vi "Teleop.vi"(10 "Match Info":T1={"Autonomous Elapsed Seconds"=0.0, "TeleOp Elapsed Seconds"=0.0, "Disabled Elapsed Seconds"=0.0, "Visited Autonomous"=FALSE, "Visited TeleOp"=FALSE, "Visited Disabled"=FALSE, "Autonomous Settings"={"Autonomous Style"=enum."Independent", "VI Refnum"=refnum}}, 11 "Call Context":T2) -> ()   [LabVIEW 2015]
doc: "This VI is called for each enabled TeleOp packet received from the DS. It is typically used to read from joysticks and other inputs and update I/O or setpoints for timed control loops. It should complete and return within 20 milliseconds or risk missing DS packets."
uses:
  <vilib>/Rock Robotics/WPI/DriverStation/WPI_DriverStationDerivedRobotMode.ctl
  <vilib>/Rock Robotics/WPI/DriverStation/WPI_DriverStationMatch Info.ctl
  <vilib>/Rock Robotics/WPI/Utilities/WPI_GetSetVariantRefNum.vi
  <vilib>/Rock Robotics/Network Tables/NT Write Boolean Array.vi
  <vilib>/Rock Robotics/Network Tables/NT Write Numeric Array.vi
  Framework/Robot Global Data.vi
  <vilib>/Rock Robotics/Network Tables/NT Write Number.vi
  <vilib>/Rock Robotics/Network Tables/NT Write Boolean.vi
panel:
  in  "Setpoint":dbl
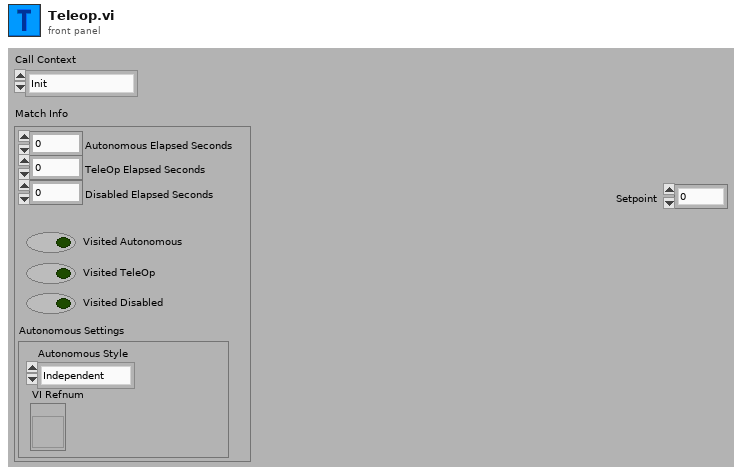
[diagram p1: front panel]
types:
  T1 = typedef "WPI_DriverStationMatch Info.ctl" = cluster{"Autonomous Elapsed Seconds":dbl, "TeleOp Elapsed Seconds":dbl, "Disabled Elapsed Seconds":dbl, "Visited Autonomous":bool, "Visited TeleOp":bool, "Visited Disabled":bool, "Autonomous Settings":cluster{"Autonomous Style":enum16{"Iterative", "Independent"}, "VI Refnum":refnum<vi>}}
  T2 = typedef "WPI_DriverStationDerivedRobotMode.ctl" = enum16{"Init", "Execute", "Stop"}
  T3 = typedef "WPI_MotorControlDeviceRef.ctl" = cluster{"DeviceStatus":errorcluster, "Type":T4, "PWM":cluster{"PWM Channel":T5, "DeadBand":T6}, "CAN":cluster{"Device Number":u8, "Control Mode":T7, "Semaphore":T8, "Max Vout":dbl, "TalonSRX Control Mode":T9}, "Invert":bool}
  T4 = typedef "WPI_MotorControlType.ctl" = enum16{"PWM", "CAN", "CANTalonSRX"}
  T5 = typedef "FPGA_DIOPWMChannel.ctl" = enum8{"PWM 0", "PWM 1", "PWM 2", "PWM 3", "PWM 4", "PWM 5", "PWM 6", "PWM 7", "PWM 8", "PWM 9", "PWM MXP 0", "PWM MXP 1", "PWM MXP 2", "PWM MXP 3", "PWM MXP 4", "PWM MXP 5", "PWM MXP 6", "PWM MXP 7", "PWM MXP 8", "PWM MXP 9", "Invalid"}
  T6 = typedef "WPI_PWMDeadband.ctl" = cluster{"Name":string, "maxPositivePwm":i32, "minPositivePwm":i32, "centerPwm":i32, "maxNegativePwm":i32, "minNegativePwm":i32, "angularRange":u16}
  T7 = typedef "WPI_CANJaguar_ControlMode.ctl" = enum8{"Percent VBus", "Current", "Speed", "Position", "Voltage"}
  T8 = typedef "Semaphore RefNum" = refnum<k1>
  T9 = typedef "WPI_CANTalonSRX_APIControlMode.ctl" = enum8{"Percent VBus", "Speed", "Position", "Slave", "Unchanged / Invalid", "Voltage Compensation", "Current", "Motion Profile"}
  T10 = typedef "WPI_CANTalonSRX_GlobalStatus.ctl" = cluster{"Applied Throttle":dbl, "Module Enabled":bool, "CAN Error":errorcluster, "Closed Loop Error":dbl, "Forward Limit Switch Closed":bool, "Reverse Limit Switch Closed":bool, "Sensor Position":dbl, "Sensor Velocity":dbl, "Current":dbl, "Sticky Fault - Over Temp":bool, "Sticky Fault - Under Voltage":bool, "Sticky Fault - Forward Limit":bool, "Sticky Fault - Reverse Limit":bool, "Sticky Fault - Forward Soft Limit":bool, "Sticky Fault - Reverse Soft Limit":bool, "Brake is Enabled":bool, "Encoder Position":dbl, "Encoder Velocity":dbl, "Encoder Index Count":dbl, "Encoder A Pin State":bool, "Encoder B Pin State":bool, "Encoder Index Pin State":bool, "Analog In":dbl, "Analog In Velocity":dbl, "Temperature (C)":dbl, "Battery Voltage":dbl, "Control 5 Is Supported":bool, "Current Profile Slot Select":dbl, "Pos Div 8":bool, "Vel Div 4":bool, "Pulse Width Position":i32, "Pulse Width Velocity":i32, "Pulse Width Rise To Rise (us)":i32, "Pulse Width Rise To Fall (us)":i32, "Mot Prof Active Is Under Run":bool, "Mot Prof Active Has Under Run":bool, "Mot Prof Active Is Last":bool, "Mot Prof Active Velocity Only":bool, "Mot Prof Active Is Valid":bool, "Mot Prof Buffer Is Full":bool, "Mot Prof Active Profile Slot Select":i32, "Mot Prof NextID":i32, "Mot Prof Count":i32, "Mot Prof Active Velocity":dbl, "Mot Prof Active Position":dbl, "Mot Prof Output Enable":i32}
  T11 = typedef "WPI_JoystickDevRef.ctl" = cluster{"Device":T12}
  T12 = typedef "WPI_JoystickDeviceEnum.ctl" = enum16{"USB 0", "USB 1", "USB 2", "USB 3", "USB 4", "USB 5"}
  T13 = typedef "WPI_AnalogChannelDevRef.ctl" = cluster{"DevStatus":errorcluster, "Analog Channel":T14}
  T14 = typedef "FPGA_AIChannel.ctl" = enum8{"AI 0", "AI 1", "AI 2", "AI 3", "AI MXP 0", "AI MXP 1", "AI MXP 2", "AI MXP 3", "Invalid"}
  T15 = typedef "WPI_CompressorDevRef.ctl" = cluster{"DevStatus":errorcluster, "Pneumatics Control Module":u8}
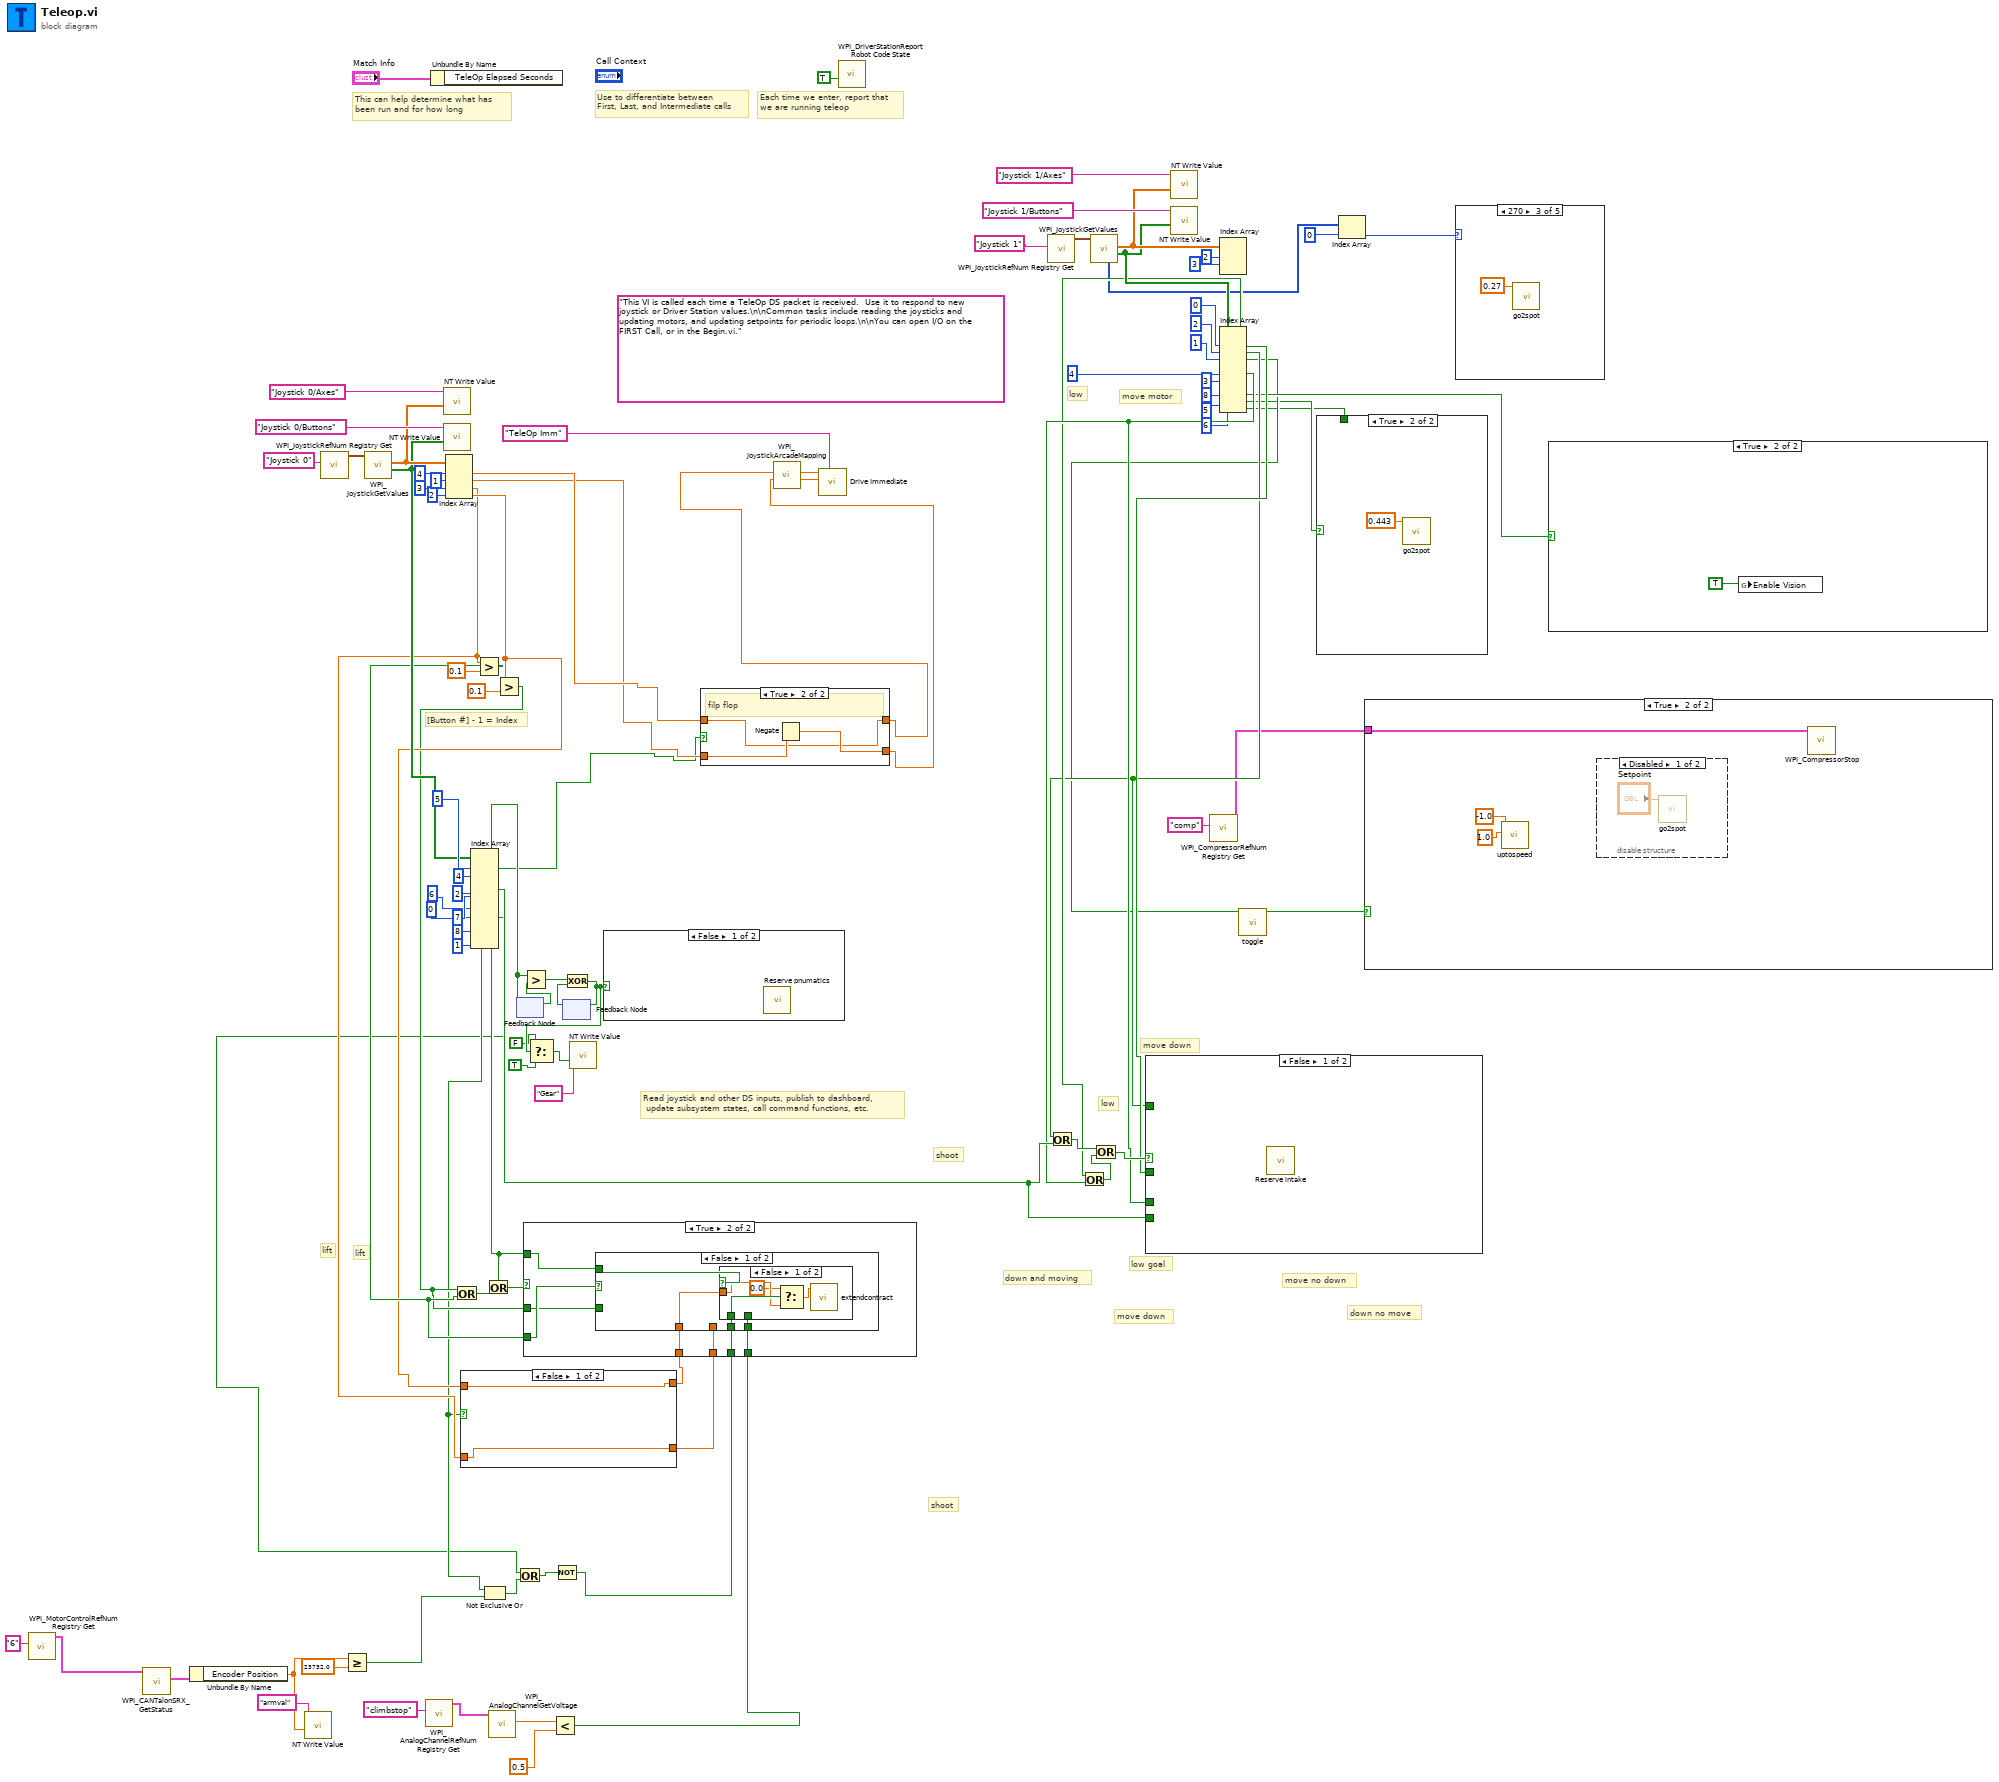
[diagram p0: block diagram]
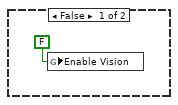
[diagram p2: hidden frame]
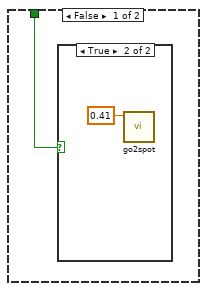
[diagram p3: hidden frame]
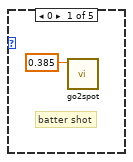
[diagram p5: hidden frame]
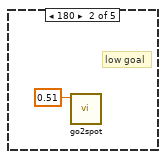
[diagram p6: hidden frame]
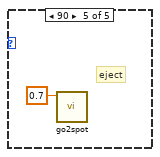
[diagram p8: hidden frame]
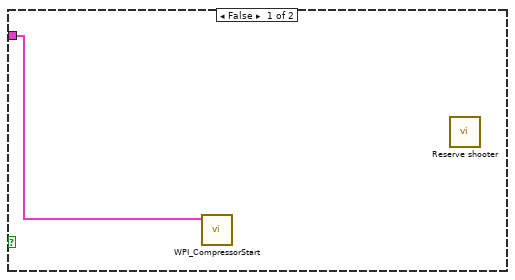
[diagram p9: hidden frame]
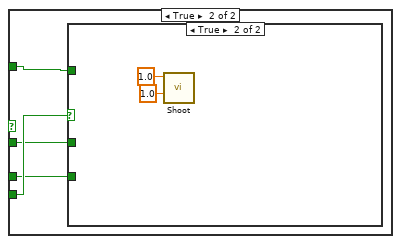
[diagram p12: hidden frame]
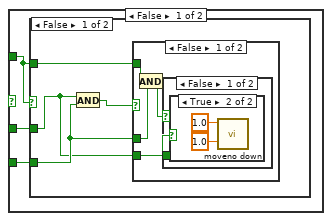
[diagram p13: hidden frame]
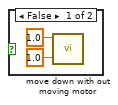
[diagram p14: hidden frame]
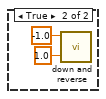
[diagram p15: hidden frame]
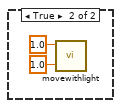
[diagram p16: hidden frame]
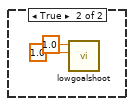
[diagram p17: hidden frame]
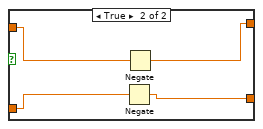
[diagram p18: hidden frame]
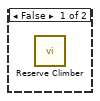
[diagram p19: hidden frame]
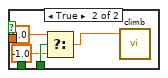
[diagram p20: hidden frame]
diagram:
  (unwired) "This VI is called each time a TeleOp DS packet is received.  Use it to respond to new joystick or Driver Station values.\n\nCommon tasks include reading the joysticks and updating motors, and updating setpoints for periodic loops.\n\nYou can open I/O on the FIRST Call, or in the Begin.vi."
  # "move down"
  # "low"
  # "down no move"
  # "move no down"
  # "shoot"
  # "low goal"
  # "down and moving"
  # "move down"
  # "shoot"
  # "move motor"
  # "low"
  # "lift"
  # "lift"
  # "[Button #] - 1 = Index"
  # "Read joystick and other DS inputs, publish to dashboard,\n update subsystem states, call command functions, etc."
  # "Each time we enter, report that\nwe are running teleop"
  # "Use to differentiate between\nFirst, Last, and Intermediate calls"
  # "This can help determine what has\nbeen run and for how long"
  n1 = call <vilib>:"WPI_MotorControlRefNum Registry Get.vi"("refnum name"="6") -> ("MotorControlDevRef"=w17:T3)  [unwired: 9 in, 1 out]
  n2 = call <vilib>:"WPI_CANTalonSRX_GetStatus.vi"("CAN Talon SRX Ref"=w17) -> ("Talon SRX Status"=w16:T10)  [unwired: 8 in, 2 out]
  n3 = Unbundle By Name(w16) -> ("Encoder Position"=w2:dbl)
  n4 = call-poly <vilib>:"NT Write Value.vi"("Numeric"=w2, "Name"="armval") -> ()  [unwired: 9 in, 1 out]
  n5 = call <vilib>:"WPI_JoystickRefNum Registry Get.vi"("refnum name"="Joystick 0") -> ("JoystickDevRef"=w95:T11)  [unwired: 1 in, 9 out]
  n6 = Greater Or Equal?(x=w2, y=23732.0) -> (x >= y?=w11:bool)
  n7 = call <vilib>:"WPI_JoystickGetValues.vi"("JoystickDevRef"=w95) -> ("Buttons"=w71:bool[], "Axes"=w92:dbl[])  [unwired: 6 in, 3 out]
  n8 = call <vilib>:"WPI_AnalogChannelRefNum Registry Get.vi"("refnum name"="climbstop") -> ("AIDeviceRef"=w4:T13)  [unwired: 9 in, 1 out]
  n9 = Unbundle By Name("Match Info") -> ()  [unwired: 1 out]
  n10 = call-poly <vilib>:"NT Write Value.vi"("Numeric Array"=w92, "Name"="Joystick 0/Axes") -> ()  [unwired: 9 in, 1 out]
  n11 = call-poly <vilib>:"NT Write Value.vi"("Boolean Array"=w71, "Name"="Joystick 0/Buttons") -> ()  [unwired: 9 in, 1 out]
  n12 = Index Array(array=w92, index #1=4 ("index"), index #2=1 ("index"), index #3=3 ("index"), index #4=2 ("index")) -> (element #1=w40:dbl, element #2=w39:dbl, element #3=w57:dbl, element #4=w58:dbl)
  n13 = Index Array(array=w71, index #1=5 ("index"), index #2=4 ("index"), index #4=2 ("index"), index #5=0 ("index"), index #6=6 ("index"), index #8=7 ("index"), index #10=8 ("index"), index #12=1 ("index")) -> (element #1=w38:bool, element #2=w75:bool, element #4=w49:bool, element #5=w60:bool, element #6=w10:bool, element #8=w8:bool)  [unwired: 4 in, 6 out]
  n14 = case shown="False" w10 {
    tunnel: [w100 w101] -> w56
    tunnel: w58 -> [w100 w104]
    tunnel: w57 -> [w99 w103]
    tunnel: [w99 w102] -> w3
    frame False {
    }
    frame True {
      n15 = Negate(x=w103) -> (-x=w102:dbl)
      n16 = Negate(x=w104) -> (-x=w101:dbl)
    }
  }
  n17 = Greater?(x=w57, y=0.1) -> (0:w63:bool)
  n18 = Not Exclusive Or(1:w11, 2:w10) -> (0:w9:bool)
  n19 = call <vilib>:"WPI_AnalogChannelGetVoltage.vi"("AIDeviceRef"=w4) -> ("Voltage"=w15:dbl)  [unwired: 8 in, 2 out]
  n20 = Greater?(x=w58, y=0.1) -> (0:w19:bool)
  n21 = Or(x=w19, y=w63) -> (x .or. y?=w61:bool)
  n22 = Or(x=w60, y=w61) -> (x .or. y?=w59:bool)
  n23 = feedback-in #1(w75) -> ()
  n24 = feedback #1() -> (w88:bool)  [unwired: 1 in]
  n25 = Or(x=w8, y=w9) -> (x .or. y?=w7:bool)
  n26 = Greater?(x=w75, y=w88) -> (0:w87:bool)
  n27 = Less?(x=w15, y=0.5 ("x")) -> (x < y?=w13:bool)
  n28 = Not(x=w7) -> (.not. x?=w6:bool)
  n29 = case shown="True" w59 {
    tunnel: w63 -> [_ w111]
    tunnel: w3 -> [_ w110]
    tunnel: w56 -> [_ w109]
    tunnel: w60 -> [_ w108]
    tunnel: w13 -> [_ w107]
    tunnel: w19 -> [_ w106]
    tunnel: w6 -> [_ w105]
    frame False {
      n30 = call "Reserve Climber.vi"() -> ()  [unwired: 11 in, 1 out]
    }
    frame True {
      n31 = case shown="False" w111 {
        tunnel: w110 -> [_ w125]
        tunnel: w109 -> [w115 w124]
        tunnel: w108 -> [w114 _]
        tunnel: w107 -> [w113 _]
        tunnel: w106 -> [_ w126]
        tunnel: w105 -> [w112 _]
        frame False {
          n32 = case shown="False" w114 {
            tunnel: w115 -> [w118 _]
            tunnel: w113 -> [_ w123]
            tunnel: w112 -> [w119 _]
            frame False {
              n33 = Select(t=0.0, s=w119, f=w118) -> (s? t:f=w116:dbl)
              n34 = call "extendcontract.vi"("Setpoint"=w116) -> ()  [unwired: 10 in, 1 out]
            }
            frame True {
              n35 = Select(t=0.0, s=w123, f=-1.0) -> (s? t:f=w120:dbl)
              n36 = call "climb.vi"("Setpoint"=w120) -> ()  [unwired: 10 in, 1 out]
            }
          }
        }
        frame True {
          n37 = case shown="True" w126 {
            tunnel: w125 -> [w127 w128]
            tunnel: w124 -> [_ w129]
            frame False {
              n38 = call "liftlower.vi"("Setpoint"=w127) -> ()  [unwired: 10 in, 1 out]
            }
            frame True {
              n39 = call "lift and contract.vi"("lift"=w128, "Setpoint"=w129) -> ()  [unwired: 9 in, 1 out]
            }
          }
        }
      }
    }
  }
  n40 = feedback #2() -> (w86:bool)  [unwired: 1 in]
  n41 = Exclusive Or(1:w86, 2:w87) -> (0:w43:bool)
  n42 = Select(t=FALSE, s=w43, f=TRUE) -> (s? t:f=w35:bool)
  n43 = feedback-in #2(w43) -> ()
  n44 = call-poly <vilib>:"NT Write Value.vi"("Boolean"=w35, "Name"="Gear") -> ()  [unwired: 9 in, 1 out]
  n45 = case shown="False" w43 {
    frame False {
      n46 = call "Reserve pnumatics.vi"() -> ()  [unwired: 11 in, 1 out]
    }
    frame True {
      n47 = call "Activate Da intake.vi"("Setpoint"=1.0) -> ()  [unwired: 10 in, 1 out]
    }
  }
  n48 = case shown="True" w38 {
    tunnel: w39 -> [w131 w135]
    tunnel: [w131 w134] -> w41
    tunnel: w40 -> [w132 w133]
    tunnel: [w132 w133] -> w42
    frame False {
    }
    frame True {
      # "filp flop"
      n49 = Negate(x=w135) -> (-x=w134:dbl)
    }
  }
  n50 = call <vilib>:"WPI_JoystickArcadeMapping.vi"("Y axis value"=w41, "X axis value"=w42) -> ("Right Motor Value"=w84:dbl, "Left Motor Value"=w85:dbl)  [unwired: 8 in]
  n51 = call "Drive Immediate.vi"("Description"="TeleOp Imm", "Right Setpoint"=w84, "Left Setpoint"=w85) -> ()  [unwired: 8 in, 1 out]
  n52 = call <vilib>:"WPI_DriverStationReport Robot Code State.vi"("TeleOp"=TRUE ("Autonomous")) -> ()  [unwired: 10 in, 1 out]
  n53 = call <vilib>:"WPI_JoystickRefNum Registry Get.vi"("refnum name"="Joystick 1") -> ("JoystickDevRef"=w81:T11)  [unwired: 1 in, 9 out]
  n54 = call <vilib>:"WPI_JoystickGetValues.vi"("JoystickDevRef"=w81) -> ("Buttons"=w72:bool[], "Axes"=w79:dbl[], "POVs"=w30:i16[])  [unwired: 6 in, 2 out]
  n55 = call-poly <vilib>:"NT Write Value.vi"("Numeric Array"=w79, "Name"="Joystick 1/Axes") -> ()  [unwired: 9 in, 1 out]
  n56 = call-poly <vilib>:"NT Write Value.vi"("Boolean Array"=w72, "Name"="Joystick 1/Buttons") -> ()  [unwired: 9 in, 1 out]
  n57 = call <vilib>:"WPI_CompressorRefNum Registry Get.vi"("refnum name"="comp") -> ("CompressorDevRef"=w31:T15)  [unwired: 9 in, 1 out]
  n58 = Index Array(array=w79, index #1=2 ("index"), index #2=3 ("index")) -> ()  [unwired: 1 in, 3 out]
  n59 = Index Array(array=w72, index #1=0 ("index"), index #2=2 ("index"), index #3=1 ("index"), index #5=4 ("index"), index #6=3 ("index"), index #8=8 ("index"), index #9=5 ("index"), index #10=6 ("index")) -> (element #1=w47:bool, element #2=w46:bool, element #3=w25:bool, element #5=w48:bool, element #8=w26:bool, element #9=w21:bool, element #10=w20:bool)  [unwired: 2 in, 3 out]
  n60 = Or(x=w46, y=w49) -> (x .or. y?=w51:bool)
  n61 = Or(x=w47, y=w48) -> (x .or. y?=w52:bool)
  n62 = Or(x=w51, y=w52) -> (x .or. y?=w50:bool)
  n63 = case shown="False" w50 {
    tunnel: w49 -> [_ w139]
    tunnel: w46 -> [_ w138]
    tunnel: w48 -> [_ w136]
    tunnel: w47 -> [_ w137]
    frame False {
      n64 = call "Reserve intake.vi"() -> ()  [unwired: 11 in, 1 out]
    }
    frame True {
      n65 = case shown="True" w139 {
        tunnel: w138 -> [w140 _]
        tunnel: w137 -> [w142 _]
        tunnel: w136 -> [w141 _]
        frame False {
          n66 = case shown="False" w140 {
            tunnel: w142 -> [w143 _]
            tunnel: w141 -> [w145 _]
            tunnel: w140 -> [w144 _]
            frame False {
              n67 = And(x=w143, y=w145) -> (x .and. y?=w146:bool)
              n68 = case shown="False" w146 {
                tunnel: w145 -> [w149 _]
                tunnel: w144 -> [w150 _]
                tunnel: w143 -> [w147 _]
                frame False {
                  n69 = And(x=w150, y=w149) -> (x .and. y?=w148:bool)
                  n70 = case shown="False" w148 {
                    tunnel: w147 -> [w151 _]
                    frame False {
                      n71 = case shown="True" w151 {
                        frame False {
                          n72 = call "move down with out moving motor.vi"("Numeric"=1.0, "Setpoint"=1.0) -> ()  [unwired: 9 in, 1 out]
                        }
                        frame True {
                          n73 = call "moveno down.vi"("Numeric"=1.0, "Setpoint"=1.0) -> ()  [unwired: 9 in, 1 out]
                        }
                      }
                    }
                    frame True {
                      n74 = call "down and reverse.vi"("Numeric"=1.0, "Setpoint"=-1.0) -> ()  [unwired: 9 in, 1 out]
                    }
                  }
                }
                frame True {
                  n75 = call "movewithlight.vi"("Numeric"=1.0, "Setpoint"=1.0) -> ()  [unwired: 9 in, 1 out]
                }
              }
            }
            frame True {
              n76 = call "lowgoalshoot.vi"("Numeric"=1.0, "Setpoint"=1.0) -> ()  [unwired: 9 in, 1 out]
            }
          }
        }
        frame True {
          n77 = call "Shoot.vi"("Numeric"=1.0, "Setpoint"=1.0) -> ()  [unwired: 9 in, 1 out]
        }
      }
    }
  }
  n78 = call "toggle.vi"("Boolean in"=w25) -> ("Boolean out"=w24:bool)  [unwired: 10 in]
  n79 = case shown="True" w21 {
    tunnel: w20 -> [w164 _]
    frame False {
      n80 = case shown="True" w164 {
        frame False {
        }
        frame True {
          n81 = call "go2spot.vi"("Setpoint"=0.41) -> ()  [unwired: 10 in, 1 out]
        }
      }
    }
    frame True {
      n82 = call "go2spot.vi"("Setpoint"=0.443) -> ()  [unwired: 10 in, 1 out]
    }
  }
  n83 = Index Array(array=w30, index=0) -> (element=w28:i16)
  n84 = case shown="True" w24 {
    tunnel: w31 -> [w167 w170]
    frame False {
      n85 = call <vilib>:"WPI_CompressorStart.vi"("CompressorDevRef"=w167) -> ()  [unwired: 9 in, 2 out]
      n86 = call "Reserve shooter.vi"() -> ()  [unwired: 11 in, 1 out]
    }
    frame True {
      n87 = call "uptospeed.vi"("on of"=1.0, "Setpoint"=-1.0) -> ()  [unwired: 9 in, 1 out]
      n88 = disable-structure shown="Disabled" {
        frame Disabled {
          n89 = call "go2spot.vi"("Setpoint"="Setpoint") -> ()  [unwired: 10 in, 1 out]
        }
        frame Enabled {
        }
      }
      n90 = call <vilib>:"WPI_CompressorStop.vi"("CompressorDevRef"=w170) -> ()  [unwired: 9 in, 2 out]
    }
  }
  n91 = case shown="270" w28 {
    frame 0 {
      # "batter shot"
      n92 = call "go2spot.vi"("Setpoint"=0.385) -> ()  [unwired: 10 in, 1 out]
    }
    frame 180 {
      # "low goal"
      n93 = call "go2spot.vi"("Setpoint"=0.51) -> ()  [unwired: 10 in, 1 out]
    }
    frame 270 {
      n94 = call "go2spot.vi"("Setpoint"=0.27) -> ()  [unwired: 10 in, 1 out]
    }
    frame -1, Default {
    }
    frame 90 {
      # "eject"
      n95 = call "go2spot.vi"("Setpoint"=0.7) -> ()  [unwired: 10 in, 1 out]
    }
  }
  n96 = case shown="True" w26 {
    frame False {
      n97 = global write "Robot Global Data.vi" "Enable Vision"(FALSE) -> ()
    }
    frame True {
      n98 = global write "Robot Global Data.vi" "Enable Vision"(TRUE) -> ()
    }
  }
